vi "Dequeue_Message_FGV.vi"(8 "error in (no error)":errorcluster, 11 "queue In":refnum<queue>) -> (0 "error out":errorcluster, 1 "Message Data":variant, 2 "Message":string)   [LabVIEW 2024, in "Relay_Module.lvlib"]
doc: "ThisVI\n------------------------------\nDequeue Message\n------------------------------\n-Dequeue the message"
uses:
  Relay_Module.lvlib
  PrivateControls/FGV_Queue_Control.ctl
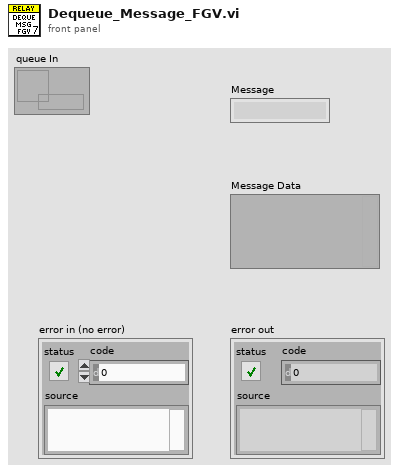
[diagram p1: front panel]
types:
  T1 = typedef "Relay_Module.lvlib/FGV_Queue_Control.ctl" = enum16{"Release", "Get", "Set"}
  T2 = cluster{"Message":string, "Message Data":variant}
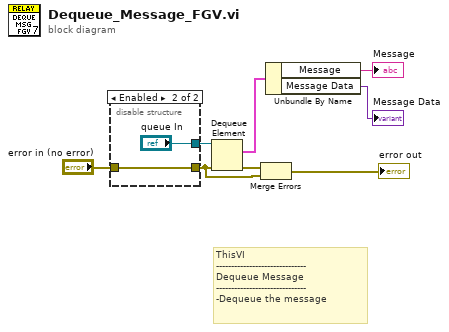
[diagram p0: block diagram]
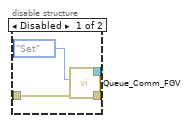
[diagram p2: hidden frame]
diagram:
  # "ThisVI\n------------------------------\nDequeue Message\n------------------------------\n-Dequeue the message"
  n1 = disable-structure shown="Enabled" {
    disable-tunnel: [w12 w14] -> w5
    disable-tunnel: [w11 "queue In"] -> w2
    disable-tunnel: "error in (no error)" -> [w10 w14]
    frame Disabled {
      n2 = call "Queue_Comm_FGV.vi"("error in (no error)"=w10, "Enum"=FGV_Queue_Control."Set") -> ("error Out"=w12:errorcluster, "queue Out"=w11:refnum<queue>)  [unwired: 8 in]
    }
    frame Enabled {
    }
  }
  n3 = Dequeue Element(queue=w2, error in (no error)=w5) -> (element=w3:T2, error out=w4:errorcluster)  [unwired: 1 in, 2 out]
  n4 = Merge Errors(w4, w5) -> (→"error out":errorcluster)
  n5 = Unbundle By Name(w3) -> ("Message"=→"Message":string, "Message Data"=→"Message Data":variant)
